vi "Read.vi"(8 "error in (no error)":errorcluster, 11 "Boolean in":refnum<class "Blackboard_Boolean.lvclass">) -> (0 "error out":errorcluster, 2 "Boolean":bool, 3 "Boolean out":refnum<class "Blackboard_Boolean.lvclass">)   [LabVIEW 2021, in "Blackboard_Boolean.lvclass"]
doc: "Abstract Data Classes 2.1.1.12\nTim Streeter - TSA\nCopyright (c) 2024, TSA"
uses:
  Blackboard_Boolean.lvclass
  Blackboard_Boolean.lvclass/Blackboard_Boolean.ctl
  Blackboard.lvclass
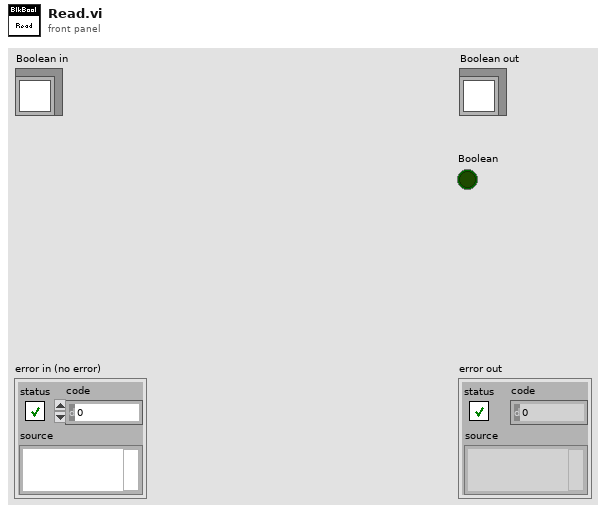
[diagram p1: front panel]
types:
  T1 = typedef "Blackboard.lvclass/Groups Type.ctl" = cluster{"Data":T2[], "Map":T5}
  T2 = typedef "Blackboard.lvclass/Data DVR Type.ctl" = cluster{"Tags":T3, "Data Refs":T4}
  T3 = typedef "Blackboard.lvclass/Tags Map Type.ctl" = map{string, refnum<class "Abs_Value.lvclass">}
  T4 = typedef "Local Bus.lvclass/Data Value References.ctl" = cluster{"Boolean":refnum<data-value>, "String":refnum<data-value>, "DBL":refnum<data-value>, "SGL":refnum<data-value>, "EXT":refnum<data-value>, "U8":refnum<data-value>, "U16":refnum<data-value>, "U32":refnum<data-value>, "U64":refnum<data-value>, "I8":refnum<data-value>, "I16":refnum<data-value>, "I32":refnum<data-value>, "I64":refnum<data-value>, "CDBL":refnum<data-value>, "CSGL":refnum<data-value>, "CEXT":refnum<data-value>, "Time":refnum<data-value>, "Variant":refnum<data-value>, "Waveform":refnum<data-value>, "Type":refnum<data-value>}
  T5 = typedef "Blackboard.lvclass/Group Map Type.ctl" = map{string, i32}
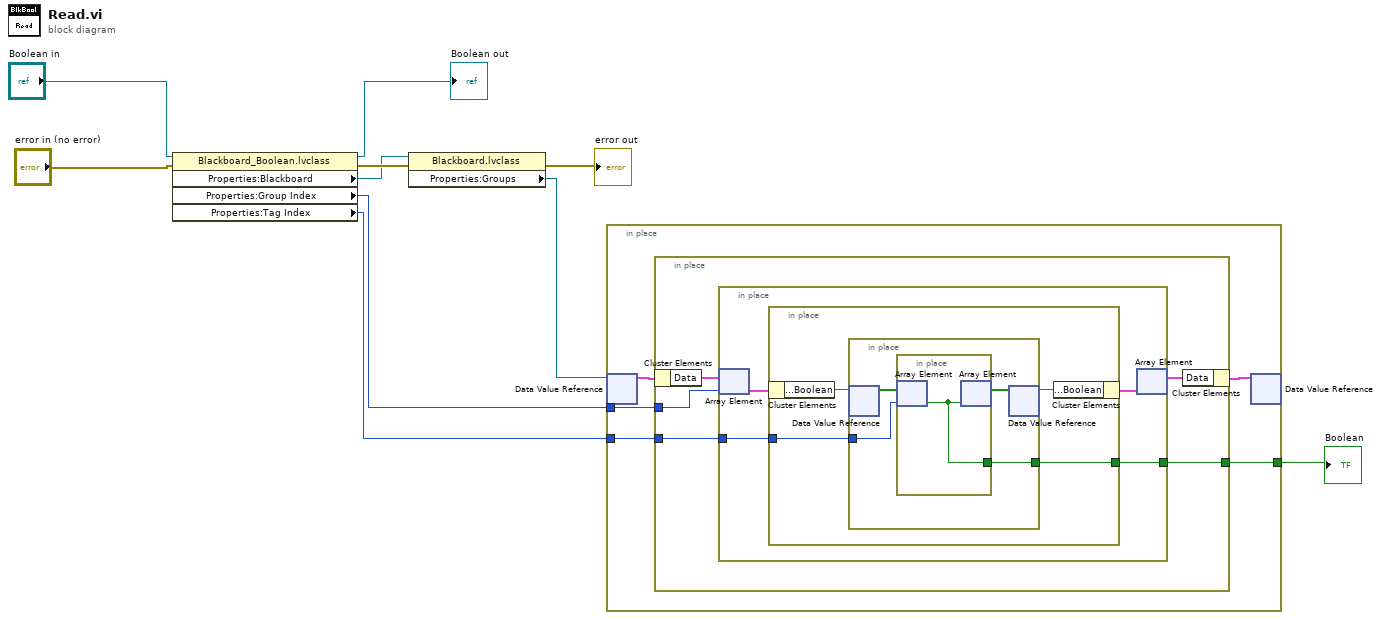
[diagram p0: block diagram]
diagram:
  n1 = property class="Blackboard_Boolean.lvclass"(reference="Boolean in", error in="error in (no error)") -> (reference out=→"Boolean out":refnum<class "Blackboard_Boolean.lvclass">, error out=w10:errorcluster, "Properties:Blackboard"=w6:refnum<class "Blackboard.lvclass">, "Properties:Group Index"=w9:i32, "Properties:Tag Index"=w7:i32)
  n2 = property class="Blackboard.lvclass"(reference=w6, error in=w10) -> (error out=→"error out":errorcluster, "Properties:Groups"=w1:refnum<data-value>)  [unwired: 1 out]
  n3 = in-place {
    in-place-border: w9 -> [w15]
    in-place-border: w7 -> [w14]
    in-place-border: [w13] -> w2
    n4 = in-place-dvr #1(w1) -> (w12:T1)  [unwired: 1 out]
    n5 = in-place {
      in-place-border: w15 -> [w20]
      in-place-border: w14 -> [w19]
      in-place-border: [w18] -> w13
      n6 = in-place-cluster #2(w12) -> ("Data"=w17:T2[])
      n7 = in-place {
        in-place-border: w19 -> [w23]
        in-place-border: [w21] -> w18
        n8 = in-place-array #3(w17, w20) -> (w24:T2)
        n9 = in-place {
          in-place-border: w23 -> [w26]
          in-place-border: [w25] -> w21
          n10 = in-place-cluster #4(w24) -> ("Data Refs.Boolean"=w28:refnum<data-value>)
          n11 = in-place {
            in-place-border: w26 -> [w30]
            in-place-border: [w29] -> w25
            n12 = in-place-dvr #5(w28) -> (w32:bool[])  [unwired: 1 out]
            n13 = in-place {
              in-place-border: [w33] -> w29
              n14 = in-place-array #6(w32, w30) -> (w33:bool)
              n15 = in-place-array #6(w33) -> (w31:bool[])  [unwired: 1 out]
            }
            n16 = in-place-dvr #5(w31) -> (w27:refnum<data-value>)  [unwired: 1 out]
          }
          n17 = in-place-cluster #4("Data Refs.Boolean"=w27) -> (w22:T2)
        }
        n18 = in-place-array #3(w22) -> (w16:T2[])  [unwired: 1 out]
      }
      n19 = in-place-cluster #2("Data"=w16) -> (w11:T1)
    }
    n20 = in-place-dvr #1(w11) -> ()  [unwired: 2 out]
  }
  "Boolean" <- w2
